vi "acquireValue.vi"(8 "error in (no error)":errorcluster, 10 "nextSample?":bool, 11 "start in":refnum<class "start.lvclass">) -> (0 "error out":errorcluster, 1 "function return":i32, 2 "variantData":variant, 3 "start out":refnum<class "start.lvclass">)   [LabVIEW 2016, in "SALLV_MtAtElectrometer_Messaging.lvlib" / "start.lvclass"]
uses:
  start.lvclass
  start.lvclass/start.ctl
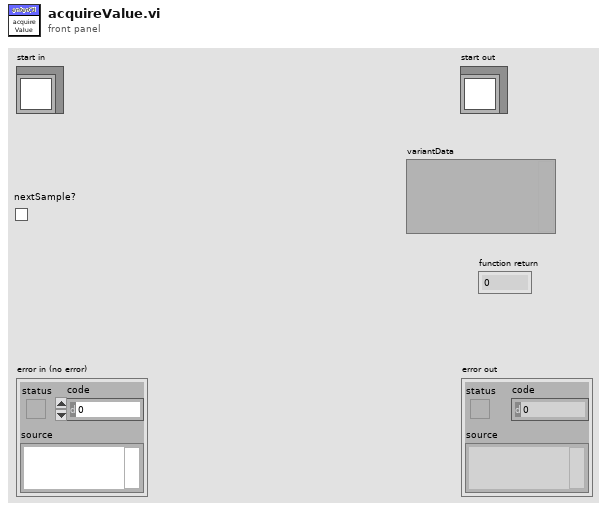
[diagram p1: front panel]
types:
  T1 = typedef "SALLV_EXA.lvlib/command_start.ctl" = cluster{"settingsToApply":string}
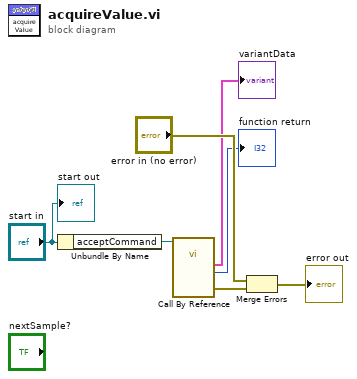
[diagram p0: block diagram]
diagram:
  n1 = Unbundle By Name("start in") -> ("acceptCommand"=w6:refnum<vi>)
  n2 = call-by-ref "?"(reference=w6) -> ("error out"=w7:errorcluster, "function return"=→"function return":i32, "command_start_Ctl out"=→"variantData":T1)  [unwired: 10 in, 2 out]
  n3 = Merge Errors("error in (no error)", w7) -> (→"error out":errorcluster)
  "start out" <- "start in"
